vi "Initialize Toolbar.vi"(7 "Background Color":u32(colorbox)=16777226, 8 "error in (no error)":errorcluster, 9 "Picture Control Bounds":T3, 10 "Vertical Icon Settings":T1={"Button Width"=32, "Button Height"=32, "Separator Height"=16}, 11 "Horizontal Icon Settings":T2={"Button Width"=64, "Button Height"=64, "Separator Width"=16, "More Options Width"=32}) -> (0 "error out":errorcluster, 3 "Toolbar Control out":refnum<class "Toolbar Control.lvclass">)   [LabVIEW 2011, in "Toolbar Control.lvclass"]
doc: "This VI will create a toolbar and return it on <B>Toolbar Control out</B>. This toolbar object can handle mouse movement, items selection and image redraw.\n\n-------------\nDeveloped by Brian Hoover (hooovahh)"
uses:
  Toolbar Control.lvclass
  <vilib>/Utility/miscctls.llb/LVRectTypeDef.ctl
  Controls/Horizontal Initialize Settings.ctl
  Controls/Vertical Initialize Settings.ctl
  Controls/Mouse State.ctl
  Controls/Button Pressed User Event Data.ctl
  Controls/Button State.ctl
  Toolbar Control.lvclass/Toolbar Control.ctl
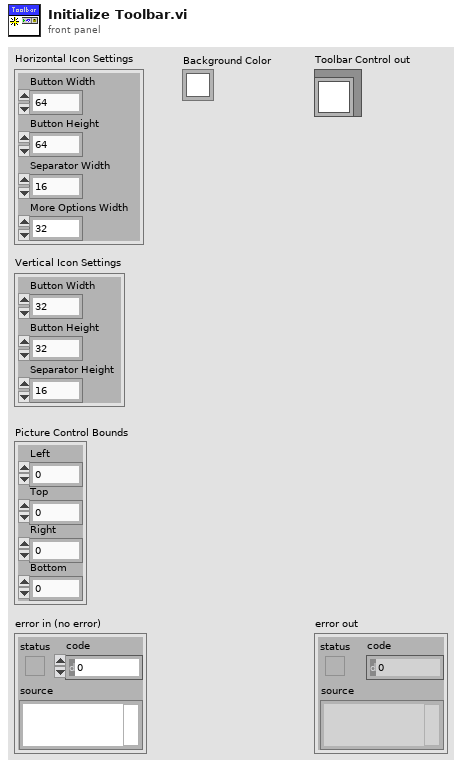
[diagram p1: front panel]
types:
  T1 = typedef "Vertical Initialize Settings.ctl" = cluster{"Button Width":i32, "Button Height":i32, "Separator Height":i32}
  T2 = typedef "Horizontal Initialize Settings.ctl" = cluster{"Button Width":i32, "Button Height":i32, "Separator Width":i32, "More Options Width":i32}
  T3 = typedef "LVRectTypeDef.ctl" = cluster{"Left":i16, "Top":i16, "Right":i16, "Bottom":i16}
  T4 = typedef "Button Pressed User Event Data.ctl" = cluster{"Button Pressed":string, "Button State":T5, "Icon Index Over":i32}
  T5 = typedef "Toolbar Control.lvclass/Button State.ctl" = enum8{"Enabled", "Disabled", "Disabled and Grayed Out"}
  T6 = typedef "Mouse State.ctl" = enum8{"Normal", "Mouse Over", "Mouse Down"}
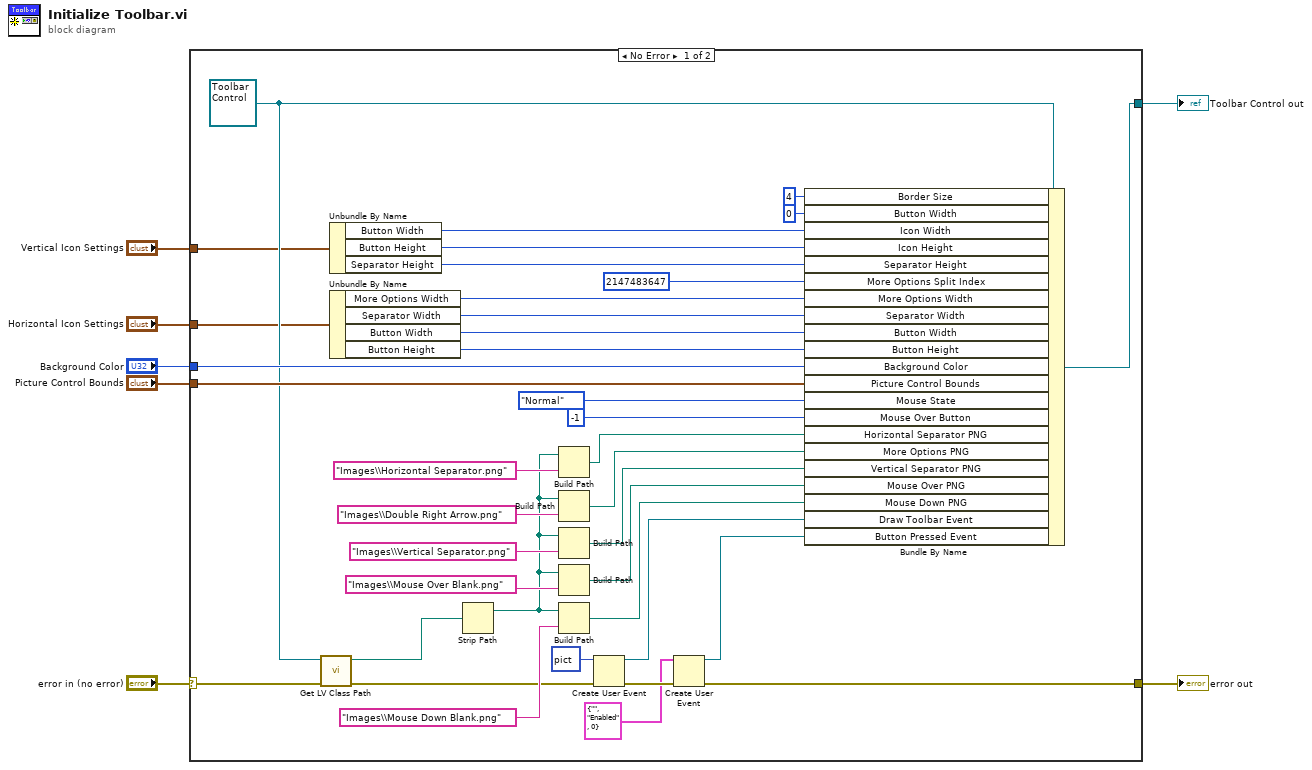
[diagram p0: block diagram]
diagram:
  n1 = case shown="No Error" "error in (no error)" {
    selector: "error in (no error)" -> [w40 w46]
    tunnel: [w22 w46] -> w6
    tunnel: [w45 _] -> w5
    tunnel: "Background Color" -> [w44 _]
    tunnel: "Picture Control Bounds" -> [w43 _]
    tunnel: "Horizontal Icon Settings" -> [w18 _]
    tunnel: "Vertical Icon Settings" -> [w13 _]
    frame No Error {
      w39 = refnum<class "Toolbar Control.lvclass"> refnum ("Toolbar Control in")
      n2 = call <vilib>:"Get LV Class Path.vi"("error in (no error)"=w40, "object"=w39) -> ("error out"=w28:errorcluster, "class path"=w38:path)  [unwired: 8 in]
      n3 = Unbundle By Name(w13) -> ("Button Width"=w12:i32, "Button Height"=w11:i32, "Separator Height"=w10:i32)
      n4 = Unbundle By Name(w18) -> ("More Options Width"=w17:i32, "Separator Width"=w16:i32, "Button Width"=w15:i32, "Button Height"=w14:i32)
      n5 = Strip Path(path=w38) -> (stripped path=w19:path)  [unwired: 1 out]
      n6 = Build Path(base path=w19, name or relative path="Images\\Horizontal Separator.png") -> (appended path=w20:path)
      n7 = Build Path(base path=w19, name or relative path="Images\\Double Right Arrow.png") -> (appended path=w30:path)
      n8 = Build Path(base path=w19, name or relative path="Images\\Vertical Separator.png") -> (appended path=w32:path)
      n9 = Build Path(base path=w19, name or relative path="Images\\Mouse Over Blank.png") -> (appended path=w34:path)
      n10 = Build Path(base path=w19, name or relative path="Images\\Mouse Down Blank.png") -> (appended path=w36:path)
      n11 = Create User Event(user event datatype=picture data[5B] ("2D Picture"), error in=w28) -> (user event=w26:refnum<user-event>, error out=w25:errorcluster)
      n12 = Create User Event(user event datatype=T4 {"Button Pressed"="", "Button State"=enum."Enabled", "Icon Index Over"=0} ("Button Pressed"), error in=w25) -> (user event=w23:refnum<user-event>, error out=w22:errorcluster)
      n13 = Bundle By Name(cluster=w39, "Border Size"=i16 4, "Button Width"=0 ("Vertical Icon Settings.Button Width"), "Icon Width"=w12, "Icon Height"=w11, "Separator Height"=w10, "More Options Split Index"=2147483647, "More Options Width"=w17, "Separator Width"=w16, "Button Width"=w15, "Button Height"=w14, "Background Color"=w44, "Picture Control Bounds"=w43, "Mouse State"=Mouse_State."Normal", "Mouse Over Button"=-1, "Horizontal Separator PNG"=w20, "More Options PNG"=w30, "Vertical Separator PNG"=w32, "Mouse Over PNG"=w34, "Mouse Down PNG"=w36, "Draw Toolbar Event"=w26, "Button Pressed Event"=w23) -> (w45:refnum<class "Toolbar Control.lvclass">)
    }
    frame Error {
    }
  }
  "error out" <- w6
  "Toolbar Control out" <- w5
